vi "Global_CMD_Shooter.vi"() -> ()   [LabVIEW 2017]
uses:
  TypeDefs/Cluster_CMD Shooter Data.ctl
  TypeDefs/ENUM_CMD Shooter Select.ctl
panel:
  in  "CMD_Shooter":T1={"Select"=enum."Manual VBus", "Wheel VBus"=0.0, "Wheel RPM"=0.0, "Hood VBus"=0.0, "Hood Position"=0.0}
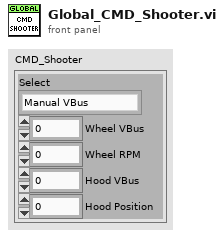
[diagram p1: front panel]
types:
  T1 = typedef "Cluster_CMD Shooter Data.ctl" = cluster{"Select":T2, "Wheel VBus":dbl, "Wheel RPM":dbl, "Hood VBus":dbl, "Hood Position":dbl}
  T2 = typedef "ENUM_CMD Shooter Select.ctl" = enum16{"Stop", "Manual VBus", "Encoder Hood Only", "Encoder Wheel Only", "Encoder Both"}
diagram:
